vi "Test SR7270.vi"() -> ()   [LabVIEW 2016, in "SR7270 Drivers.lvclass"]
uses:
  SR7270 Drivers.lvclass
  <vilib>/addons/_JKI Toolkits/Caraya/classes/Test/Test.lvclass
panel:
  out "error out":errorcluster
  in  "Serial Number":string="09337296"
  # "Test SR7270 Drivers"
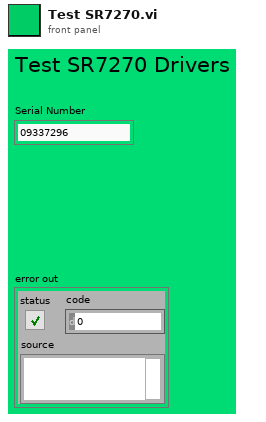
[diagram p1: front panel]
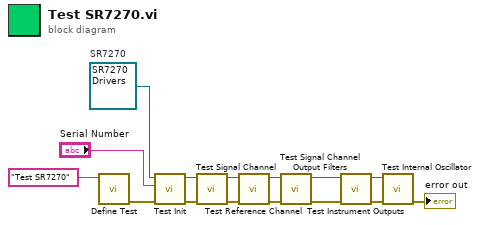
[diagram p0: block diagram]
diagram:
  w15 = refnum<class "SR7270 Drivers.lvclass"> refnum  # SR7270
  n1 = call <vilib>:"Define Test.vi"("Label (VI Title)"="Test SR7270") -> ("error out"=w12:errorcluster)  [unwired: 10 in]
  n2 = call "Test Init.vi"("error in (no error)"=w12, "Serial Number"="Serial Number", "SR7270 Drivers in"=w15) -> ("error out"=w11:errorcluster, "SR7270 Drivers out"=w10:refnum<class "SR7270 Drivers.lvclass">)  [unwired: 7 in]
  n3 = call "Test Signal Channel.vi"("error in (no error)"=w11, "SR7270 Drivers in"=w10) -> ("error out"=w9:errorcluster, "SR7270 Drivers out"=w8:refnum<class "SR7270 Drivers.lvclass">)  [unwired: 8 in]
  n4 = call "Test Reference Channel.vi"("error in (no error)"=w9, "SR7270 Drivers in"=w8) -> ("error out"=w6:errorcluster, "SR7270 Drivers out"=w7:refnum<class "SR7270 Drivers.lvclass">)  [unwired: 8 in]
  n5 = call "Test Signal Channel Output Filters.vi"("error in (no error)"=w6, "SR7270 Drivers in"=w7) -> ("error out"=w4:errorcluster, "SR7270 Drivers out"=w5:refnum<class "SR7270 Drivers.lvclass">)  [unwired: 8 in]
  n6 = call "Test Instrument Outputs.vi"("error in (no error)"=w4, "SR7270 Drivers in"=w5) -> ("error out"=w2:errorcluster, "SR7270 Drivers out"=w3:refnum<class "SR7270 Drivers.lvclass">)  [unwired: 8 in]
  n7 = call "Test Internal Oscillator.vi"("error in (no error)"=w2, "SR7270 Drivers in"=w3) -> ("error out"=→"error out":errorcluster)  [unwired: 8 in, 1 out]
